vi "Miniquads.SetVoltage.vi"(0 "i ref in":refnum<vi>, 1 "Object":string="SimChannel01", 2 "SetVoltage":dbl, 3 "ms timeout (10000)":i32=10000, 5 "error in (no error)":errorcluster) -> (14 "i ref out":refnum<vi>, 17 "timed out":bool, 19 "error out":errorcluster)   [LabVIEW 2014, in "Miniquads.lvlib"]
doc: "Writes the voltage to the object"
uses:
  Miniquads.lvlib
  CSCore/CSSystem/CoreDefs/CoreDefs.call_type.ctl
  CSCore/BaseProcess/BaseProcess.descriptor string definition.ctl
  CSCore/CSSystem/CoreDefs/CoreDefs.rawDataType.ctl
  CSCore/CSSystem/CoreLib/CoreLib.double 2 byte array.vi
  CSCore/BaseProcess/BaseProcess.lvlib
  CSCore/CSSystem/CoreLib/CoreLib.lvlib
panel:
  in  "call cluster type":T1={"Object"="", "Selector"="", "CallType"=enum."synchronous", "Async Object"="", "Async Selector"="", "Data Descriptor"="", "Data"=[], "Error #"=0, "Expire"=0}
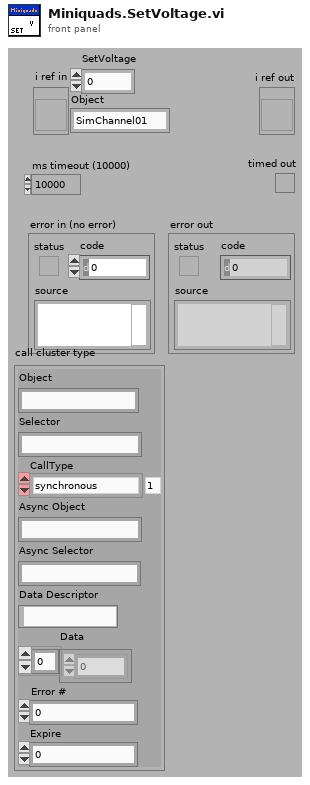
[diagram p1: front panel]
types:
  T1 = typedef "CoreDefs.call_type.ctl" = cluster{"Object":string, "Selector":string, "CallType":enum16{"simple", "synchronous", "asynchronous"}, "Async Object":string, "Async Selector":string, "Data Descriptor":T2, "Data":T3, "Error #":i32, "Expire":u32}
  T2 = typedef "BaseProcess.lvlib/BaseProcess.descriptor string definition.ctl" = string
  T3 = typedef "CoreDefs.rawDataType.ctl" = i8[]
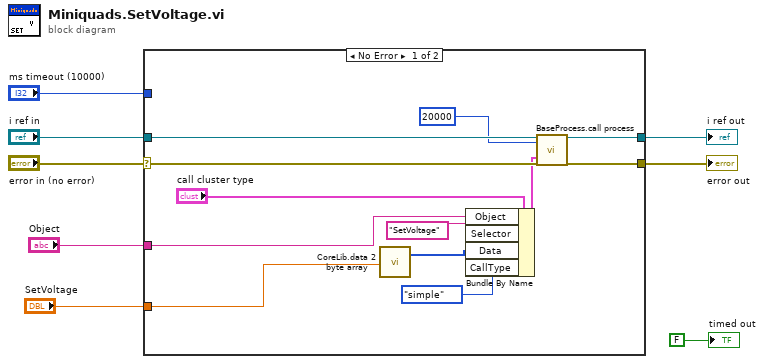
[diagram p0: block diagram]
diagram:
  n1 = case shown="No Error" "error in (no error)" {
    selector: "error in (no error)" -> [w17 w21]
    tunnel: "i ref in" -> [w18 w22]
    tunnel: [w13 w22] -> w7
    tunnel: [w12 w21] -> w5
    tunnel: "ms timeout (10000)" -> [_ _]
    tunnel: "SetVoltage" -> [w14 _]
    tunnel: "Object" -> [w11 _]
    frame No Error {
      n2 = call-poly "CoreLib.data 2 byte array.vi"("f64"=w14) -> ("byteArray out"=w19:T3)  [unwired: 18 in]
      n3 = Bundle By Name(cluster="call cluster type", "Object"=w11, "Selector"="SetVoltage", "Data"=w19, "CallType"=enum16{"simple", "synchronous", "asynchronous"}."simple") -> (w15:T1)
      n4 = call "BaseProcess.call process.vi"("i ref in"=w18, "timeout (ms)"=20000, "call cluster in"=w15, "error in (no error)"=w17) -> ("i ref out"=w13:refnum<vi>, "error out"=w12:errorcluster)  [unwired: 13 in, 1 out]
    }
    frame Error {
    }
  }
  "error out" <- w5
  "i ref out" <- w7
  "timed out" <- FALSE ("timed out")
